vi "LOG_pp3c_STATE.vi"(8 "Log memo?":bool, 10 "queue in":refnum<queue>, 11 "State In":T1={"Curr  tr"=0, "Curr (ms)"=0, "Cum (ms)"=0, "Run loop diff"=0, "Tone countdown (ms)"=0, "Countdown (ms)"=0, "Curr State"=enum."0 NULL", "Prev State"=enum."1 Habituation", "Rw"=FALSE, "Sw"=FALSE, "Tone\nGate"=FALSE, "Punish"=FALSE, "Current DAQ DO Int"=0, "Current Loaded Trial"={"Trial Type Number"=1, "Trial Type"=enum."GO", "Trial Weight"=100, "Shock (mA)"=0.3, "Duration (ms)"=0.25, "Sound Type"=enum."04 FM Sweep", "Stim P1"=4000.0, "Stim P2"=0.0, "Stim P3"=0.0, "Stim P4"=2000.0, "DAQ Amplitude (V)"=0.25}, "Total trials memo"=0, "State start cum memo (ms)"=0, "Last dur jump time memo (ms)"=0, "Last dur shock time memo (ms)"=0, "Tone repeat memo (ms)"=0, "Webcam on"=FALSE, "Webcam recording"=FALSE, "State update flag"=FALSE, "Last loaded shock voltage"=0.0, "Vid upd"=enum."0", "First time tone"=FALSE} {"Current DAQ DO Int" format="%016b"; "Current Loaded Trial"."DAQ Amplitude (V)" min=0.0 max=5.0 format="%_4g"; "Current Loaded Trial"."Shock (mA)" min=-1.0 max=5.0; "Current Loaded Trial"."Trial Weight" step=1; "Current Loaded Trial"."Duration (ms)" min=0.0 max=1.0; "Current Loaded Trial"."Trial Type Number" min=1 max=256 step=1}) -> (2 "queue out":refnum<queue>)   [LabVIEW 2013]
uses:
  CTL_pp3g_LoopState.ctl
  pp3_CTL_BehavioralState.ctl
  CTL_pp3g_Trial.ctl
  pp3_CTL_TrialType.ctl
  labolabo2/waveforms/WFTypes.ctl
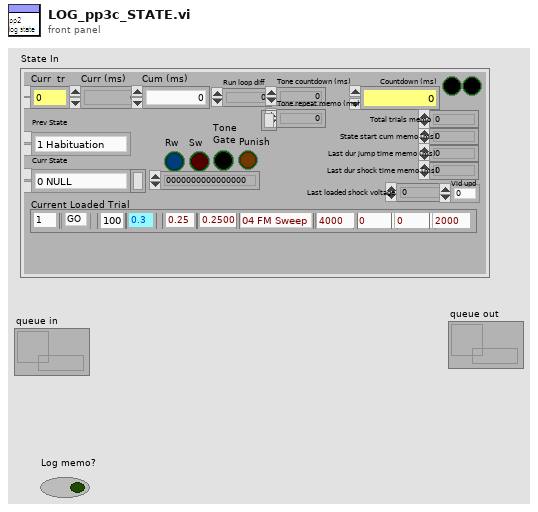
[diagram p1: front panel]
types:
  T1 = typedef "CTL_pp3g_LoopState.ctl" = cluster{"Curr  tr":u16, "Curr (ms)":u32, "Cum (ms)":u64, "Run loop diff":i64, "Tone countdown (ms)":i64, "Countdown (ms)":i64, "Curr State":T2, "Prev State":T2, "Rw":bool, "Sw":bool, "Tone\nGate":bool, "Punish":bool, "Current DAQ DO Int":u16, "Current Loaded Trial":T3, "Total trials memo":i64, "State start cum memo (ms)":i64, "Last dur jump time memo (ms)":i64, "Last dur shock time memo (ms)":i64, "Tone repeat memo (ms)":i64, "Webcam on":bool, "Webcam recording":bool, "State update flag":bool, "Last loaded shock voltage":dbl, "Vid upd":enum16{"0", "1", "2", "3", "4", "5", "6", "7", "8", "9"}, "First time tone":bool}
  T2 = typedef "pp3_CTL_BehavioralState.ctl" = enum8{"0 NULL", "1 Habituation", "2 (Load Trial)", "3 Stay Period", "4 Load Audio/Click Delay", "5 GO Trial", "6 GO Jumped", "7 GO Timeout", "8 NOGO Trial", "9 NOGO Jumped", "10 NOGO Timeout", "11 TEST Trial", "12 TEST Jumped", "13 TEST Timeout", "14 Intertrial Interval", "15 Done"}
  T3 = typedef "CTL_pp3g_Trial.ctl" = cluster{"Trial Type Number":i16, "Trial Type":T4, "Trial Weight":u32, "Shock (mA)":dbl, "Duration (ms)":dbl, "Sound Type":T5, "Stim P1":dbl, "Stim P2":dbl, "Stim P3":dbl, "Stim P4":dbl, "DAQ Amplitude (V)":dbl}
  T4 = typedef "pp3_CTL_TrialType.ctl" = enum16{"OFF", "GO", "NOGO", "TEST"}
  T5 = typedef "WFTypes.ctl" = enum16{"00 NULL", "01 DC", "02 Noise", "03 Pure Tone", "04 FM Sweep", "05 FM Sweep BURST"}
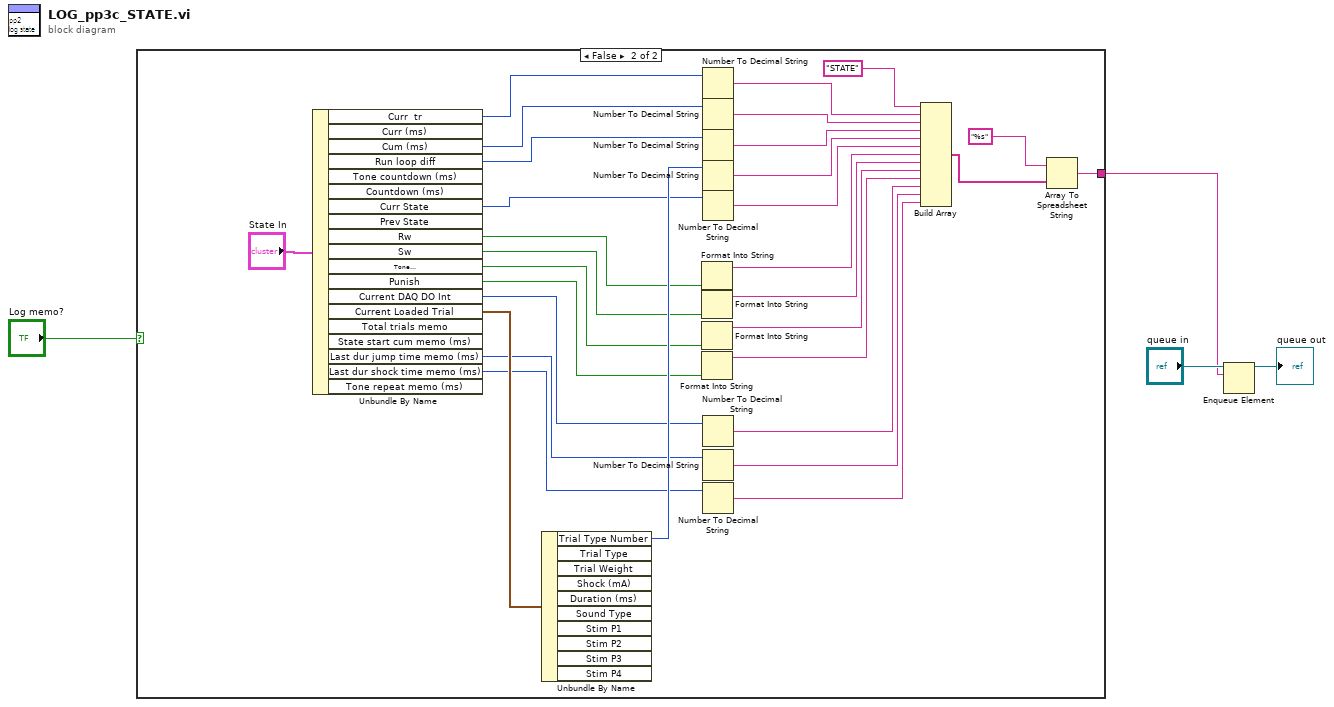
[diagram p0: block diagram]
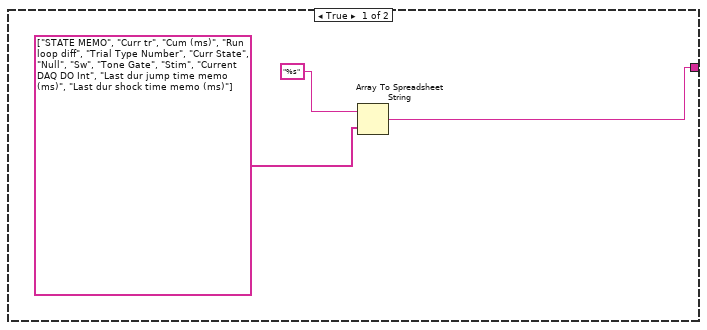
[diagram p2: hidden frame]
diagram:
  n1 = case shown="False" "Log memo?" {
    tunnel: [w5 w30] -> w1
    frame True {
      n2 = Array To Spreadsheet String(array=string[] ["STATE MEMO", "Curr tr", "Cum (ms)", "Run loop diff", "Trial Type Number", "Curr State", "Null", "Sw", "Tone Gate", "Stim", "Current DAQ DO Int", "Last dur jump time memo (ms)", "Last dur shock time memo (ms)"], 3:"%s" ("format string")) -> (spreadsheet string=w5:string)  [unwired: 1 in]
    }
    frame False {
      n3 = Unbundle By Name("State In") -> ("Curr  tr"=w27:u16, "Cum (ms)"=w26:u64, "Run loop diff"=w25:i64, "Curr State"=w22:T2, "Rw"=w21:bool, "Sw"=w20:bool, "Tone\nGate"=w19:bool, "Punish"=w18:bool, "Current DAQ DO Int"=w10:u16, "Current Loaded Trial"=w24:T3, "Last dur jump time memo (ms)"=w15:i64, "Last dur shock time memo (ms)"=w14:i64)  [unwired: 7 out]
      n4 = Unbundle By Name(w24) -> ("Trial Type Number"=w23:i16)  [unwired: 9 out]
      n5 = Format Into String(w21) -> (resulting string=w9:string)  [unwired: 3 in, 1 out]
      n6 = Format Into String(w20) -> (resulting string=w8:string)  [unwired: 3 in, 1 out]
      n7 = Format Into String(w19) -> (resulting string=w17:string)  [unwired: 3 in, 1 out]
      n8 = Format Into String(w18) -> (resulting string=w16:string)  [unwired: 3 in, 1 out]
      n9 = Number To Decimal String(number=w27) -> (decimal integer string=w28:string)  [unwired: 1 in]
      n10 = Number To Decimal String(number=w26) -> (decimal integer string=w36:string)  [unwired: 1 in]
      n11 = Number To Decimal String(number=w25) -> (decimal integer string=w35:string)  [unwired: 1 in]
      n12 = Number To Decimal String(number=w23) -> (decimal integer string=w34:string)  [unwired: 1 in]
      n13 = Number To Decimal String(number=w22) -> (decimal integer string=w33:string)  [unwired: 1 in]
      n14 = Number To Decimal String(number=w10) -> (decimal integer string=w11:string)  [unwired: 1 in]
      n15 = Number To Decimal String(number=w15) -> (decimal integer string=w13:string)  [unwired: 1 in]
      n16 = Number To Decimal String(number=w14) -> (decimal integer string=w12:string)  [unwired: 1 in]
      n17 = Build Array("STATE" ("element"), w28, w36, w35, w34, w33, w9, w8, w17, w16, w11, w13, w12) -> (w31:string[])
      n18 = Array To Spreadsheet String(array=w31, 3:"%s" ("format string")) -> (spreadsheet string=w30:string)  [unwired: 1 in]
    }
  }
  n19 = Enqueue Element(queue="queue in", element=w1) -> (queue out=→"queue out":refnum<queue>)  [unwired: 2 in, 2 out]
